vi "Prime BSI Initialize Camera.vi"(0 "Camera Index":i32, 7 "Image Ref":T1, 11 "Error In":errorcluster) -> (2 "Library Ref":refnum<k24>, 4 "Camera Ref":refnum<k24>, 13 "Camera Name":string, 15 "Error Out":errorcluster)   [LabVIEW 2020]
uses:
  <vilib>/vision/Image Controls.llb/IMAQ Image.ctl
  Camera Controls/Camera IMAQ Key Info.ctl
  Y:/Software/Photometrics/Photometrics LabView Package 2021/Dependencies/PVCamNET.dll
panel:
  out "Cooler Name":string
  out "Cooler Available":bool
  in  "Debug Mode":bool
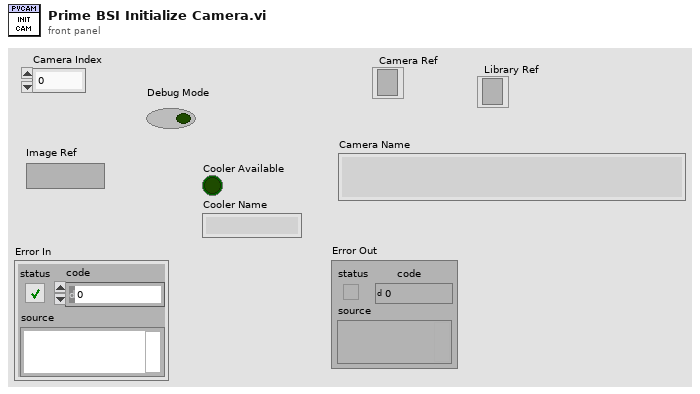
[diagram p1: front panel]
types:
  T1 = typedef "IMAQ Image.ctl" = refnum<image>
  T2 = typedef "Camera IMAQ Key Info.ctl" = cluster{"Frame":u32, "Sensor Height":i32, "Sensor Width":i32, "ROI Height":i32, "ROI Width":i32, "ROI Enable?":bool, "Bit per Pixel":u8}
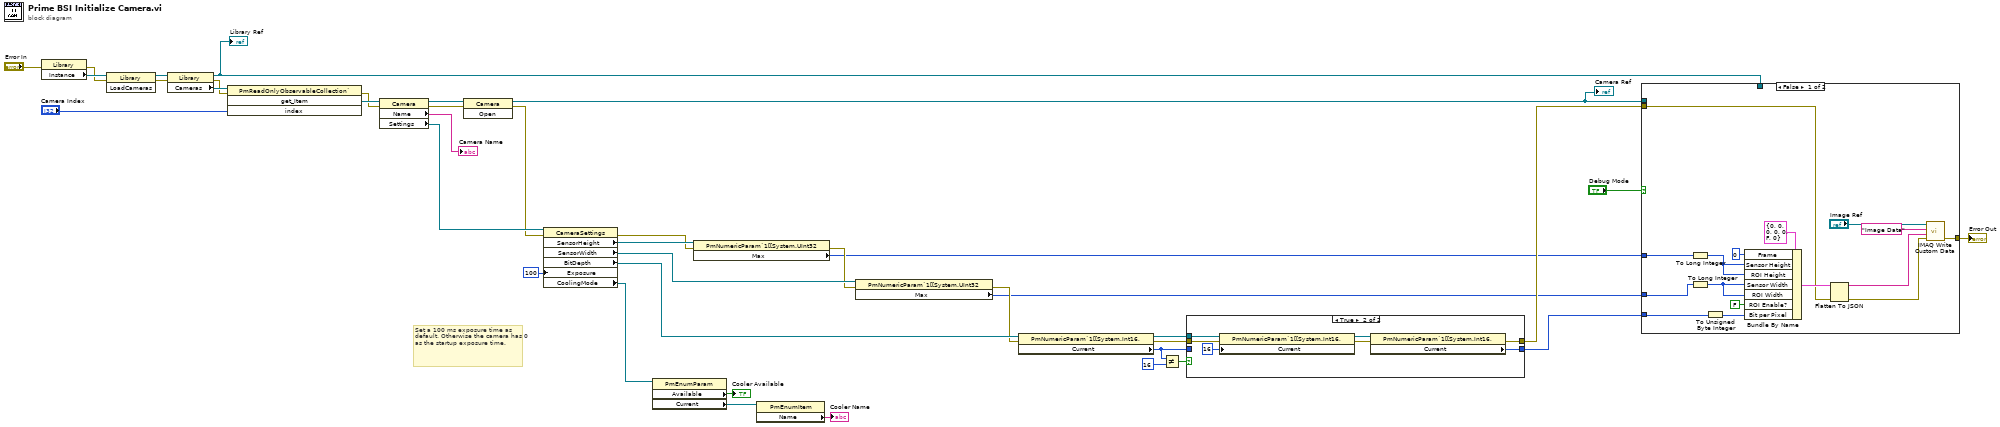
[diagram p0: block diagram]
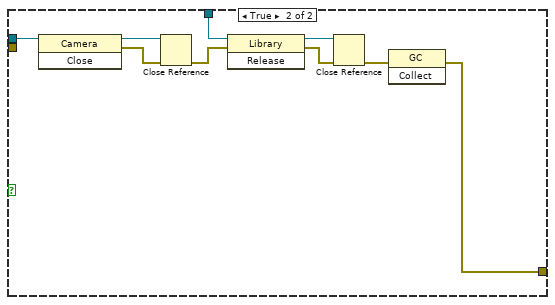
[diagram p2: hidden frame]
diagram:
  # "Set a 100 ms exposure time as default. Otherwise the camera has 0 as the startup exposure time."
  n1 = property class="Library"(error in="Error In") -> (error out=w36:errorcluster, "Instance"=w39:refnum<k24>)  [unwired: 1 in, 1 out]
  n2 = invoke class="Library" method="LoadCameras"(reference=w39, error in=w36) -> (reference out=w38:refnum<k24>, error out=w35:errorcluster)  [unwired: 1 in, 1 out]
  n3 = property class="Library"(reference=w38, error in=w35) -> (reference out=w21:refnum<k24>, error out=w34:errorcluster, "Cameras"=w37:refnum<k24>)
  "Library Ref" <- w21
  n4 = invoke class="PmReadOnlyObservableCollection`" method="get_Item"(reference=w37, error in=w34, "index"="Camera Index") -> (error out=w32:errorcluster, "get_Item"=w33:refnum<k24>)  [unwired: 1 in, 2 out]
  n5 = property class="Camera"(reference=w33, error in=w32) -> (reference out=w28:refnum<k24>, error out=w19:errorcluster, "Name"=→"Camera Name":string, "Settings"=w31:refnum<k24>)
  n6 = invoke class="Camera" method="Open"(reference=w28, error in=w19) -> (reference out=w18:refnum<k24>, error out=w17:errorcluster)  [unwired: 1 in, 1 out]
  "Camera Ref" <- w18
  n7 = property class="CameraSettings"(reference=w31, error in=w17, "Exposure"=u32 100) -> (error out=w14:errorcluster, "SensorHeight"=w16:refnum<k24>, "SensorWidth"=w15:refnum<k24>, "BitDepth"=w12:refnum<k24>, "CoolingMode"=w4:refnum<k24>)  [unwired: 1 out]
  n8 = property class="PmEnumParam"(reference=w4) -> ("Available"=→"Cooler Available":bool, "Current"=w3:refnum<k24>)  [unwired: 1 in, 2 out]
  n9 = property class="PmNumericParam`1[[System.UInt32"(reference=w16, error in=w14) -> (error out=w13:errorcluster, "Max"=w8:u32)  [unwired: 1 out]
  n10 = property class="PmEnumItem"(reference=w3) -> ("Name"=→"Cooler Name":string)  [unwired: 1 in, 2 out]
  n11 = property class="PmNumericParam`1[[System.UInt32"(reference=w15, error in=w13) -> (error out=w11:errorcluster, "Max"=w7:u32)  [unwired: 1 out]
  n12 = property class="PmNumericParam`1[[System.Int16,"(reference=w12, error in=w11) -> (reference out=w24:refnum<k24>, error out=w23:errorcluster, "Current"=w20:i16)
  n13 = Not Equal?(x=w20, y=i16 16) -> (x != y?=w25:bool)
  n14 = case shown="True" w25 {
    tunnel: w24 -> [_ w48]
    tunnel: w23 -> [w41 w47]
    tunnel: [w41 w43] -> w10
    tunnel: [w40 w42] -> w9
    tunnel: w20 -> [w40 _]
    frame False {
    }
    frame True {
      n15 = property class="PmNumericParam`1[[System.Int16,"(reference=w48, error in=w47, "Current"=i16 16) -> (reference out=w45:refnum<k24>, error out=w44:errorcluster)
      n16 = property class="PmNumericParam`1[[System.Int16,"(reference=w45, error in=w44) -> (error out=w43:errorcluster, "Current"=w42:i16)  [unwired: 1 out]
    }
  }
  n17 = case shown="False" "Debug Mode" {
    tunnel: w18 -> [_ w67]
    tunnel: w21 -> [_ w66]
    tunnel: w9 -> [w53 _]
    tunnel: w10 -> [w52 _]
    tunnel: w8 -> [w51 _]
    tunnel: w7 -> [w50 _]
    tunnel: [w49 w65] -> w6
    frame False {
      n18 = To Long Integer(number=w51) -> (32bit integer=w62:i32)
      n19 = To Long Integer(number=w50) -> (32bit integer=w63:i32)
      n20 = To Unsigned Byte Integer(number=w53) -> (unsigned 8bit integer=w61:u8)
      n21 = Bundle By Name(cluster=T2 {"Frame"=0, "Sensor Height"=0, "Sensor Width"=0, "ROI Height"=0, "ROI Width"=0, "ROI Enable?"=FALSE, "Bit per Pixel"=0} ("Camera IMAQ Key Info"), "Frame"=u32 0, "Sensor Height"=w62, "ROI Height"=w62, "Sensor Width"=w63, "ROI Width"=w63, "ROI Enable?"=FALSE, "Bit per Pixel"=w61) -> (w58:T2)
      n22 = Flatten To JSON(anything=w58, error in (no error)=w52) -> (JSON string=w59:string, 11:w64:errorcluster)  [unwired: 1 in]
      n23 = call "IMAQ Write Custom Data"("error in (no error)"=w64, "Custom Data In"=w59, "Key"="Image Data", "Image"="Image Ref") -> ("error out"=w49:errorcluster)  [unwired: 6 in, 1 out]
    }
    frame True {
      n24 = invoke class="Camera" method="Close"(reference=w67) -> (reference out=w71:refnum<k24>, error out=w69:errorcluster)  [unwired: 2 in, 1 out]
      n25 = Close Reference(reference=w71, error in (no error)=w69) -> (error out=w68:errorcluster)
      n26 = invoke class="Library" method="Release"(reference=w66, error in=w68) -> (reference out=w70:refnum<k24>, error out=w73:errorcluster)  [unwired: 1 in, 1 out]
      n27 = Close Reference(reference=w70, error in (no error)=w73) -> (error out=w72:errorcluster)
      n28 = invoke class="GC" method="Collect"(error in=w72) -> (error out=w65:errorcluster)  [unwired: 2 in, 2 out]
    }
  }
  "Error Out" <- w6
